vi "Async Data Logger.vi"(8 "error in (no error)":errorcluster, 10 "Log File Ref.":refnum<file>, 11 "User Event In":refnum<user-event>) -> (0 "error out":errorcluster)   [LabVIEW 2024, in "devicePowerSequencerCoreLogic.lvlib"]
doc: "<b> Asynchronous Logger </b> logs the measured data as they are generated. Runs independent of core logic.."
uses:
  devicePowerSequencerCoreLogic.lvlib
  dataLogger/dataLogger.lvlib
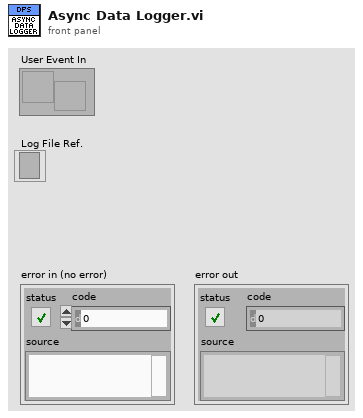
[diagram p1: front panel]
types:
  T1 = cluster{"Measured Data":cluster{"Voltage":dbl[], "Current":dbl[]}[], "Measurment Size":i32[], "Log File Ref.":refnum<file>, "First Call?":bool, "Measure Complete?":bool}
  T2 = enum16{"open", "replace", "create", "open or create", "replace or create", "replace or create with confirmation"}
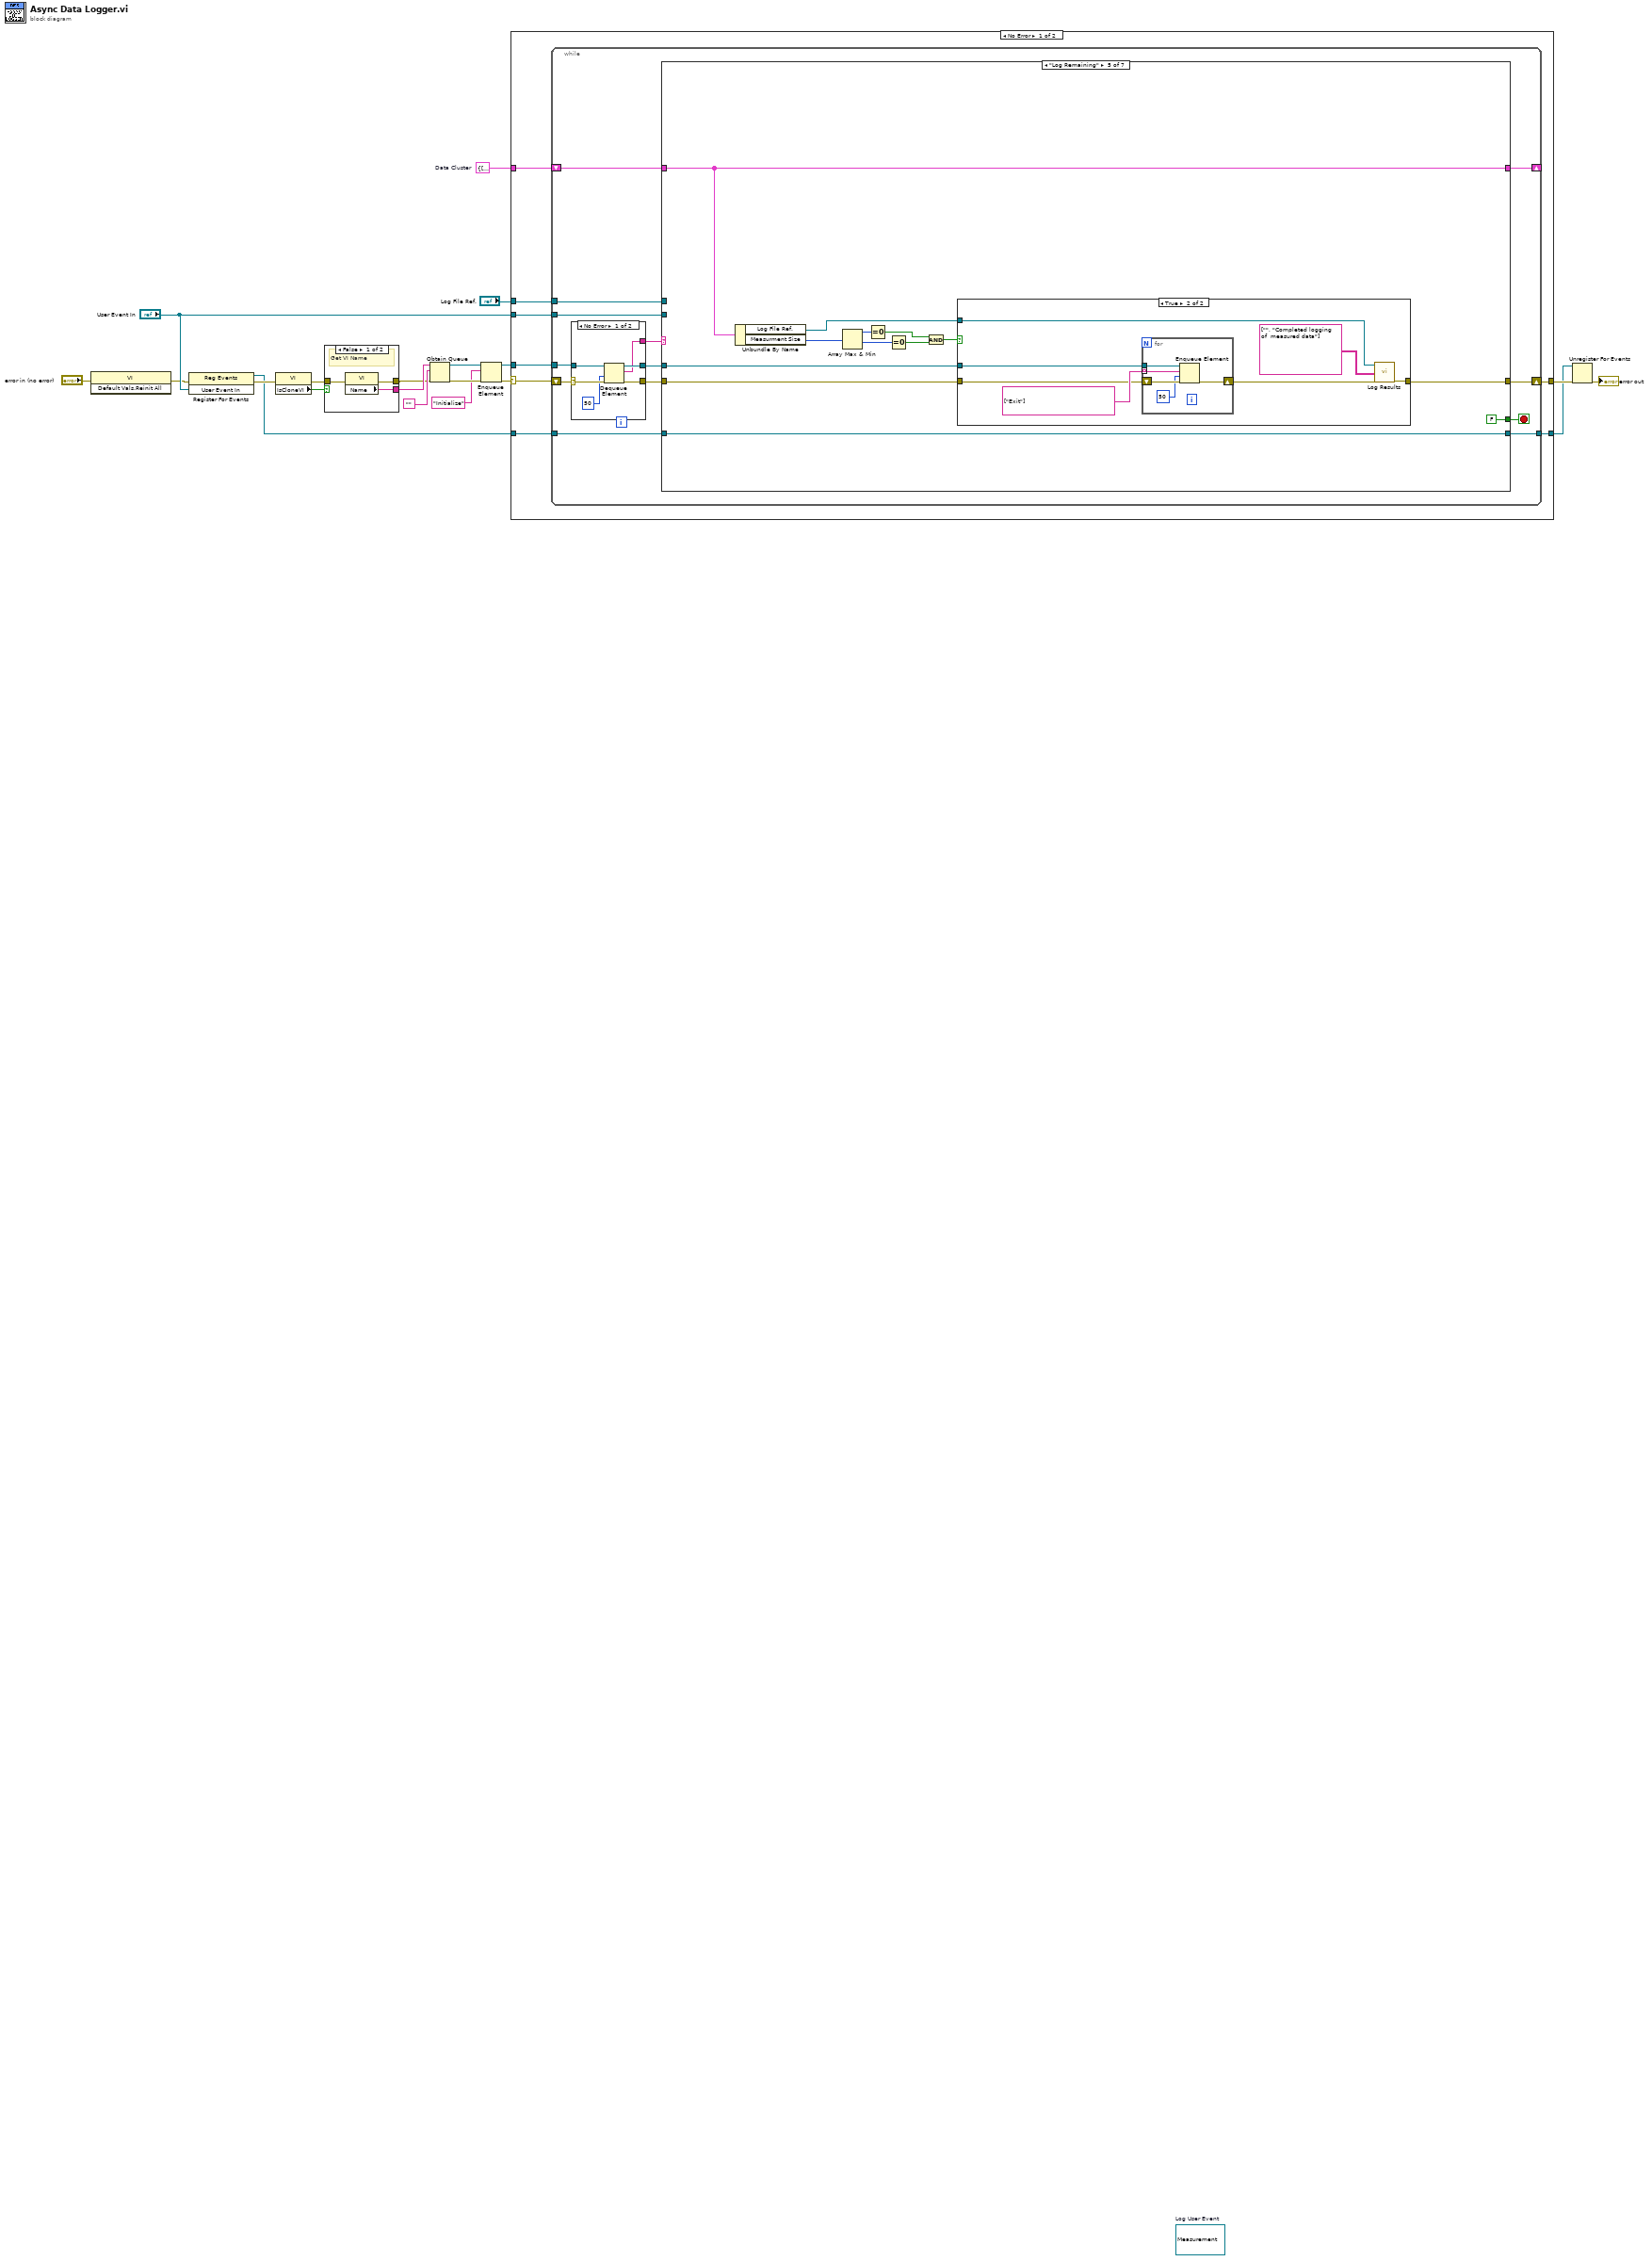
[diagram p0: block diagram]
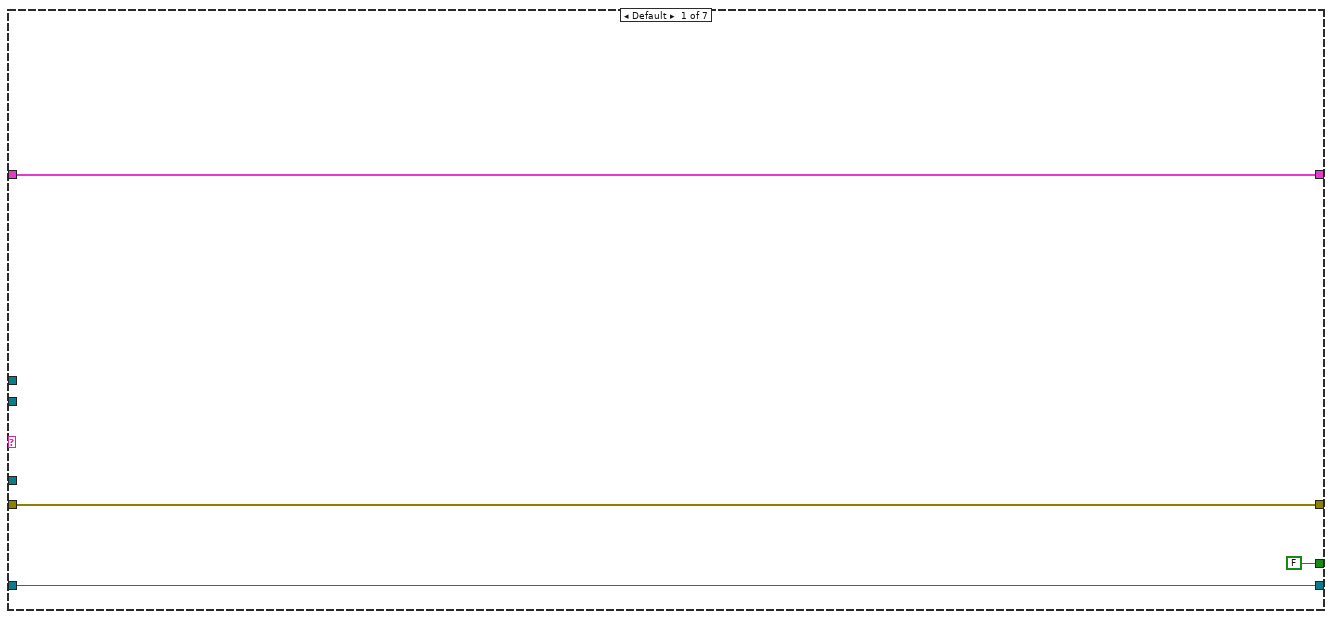
[diagram p2: hidden frame]
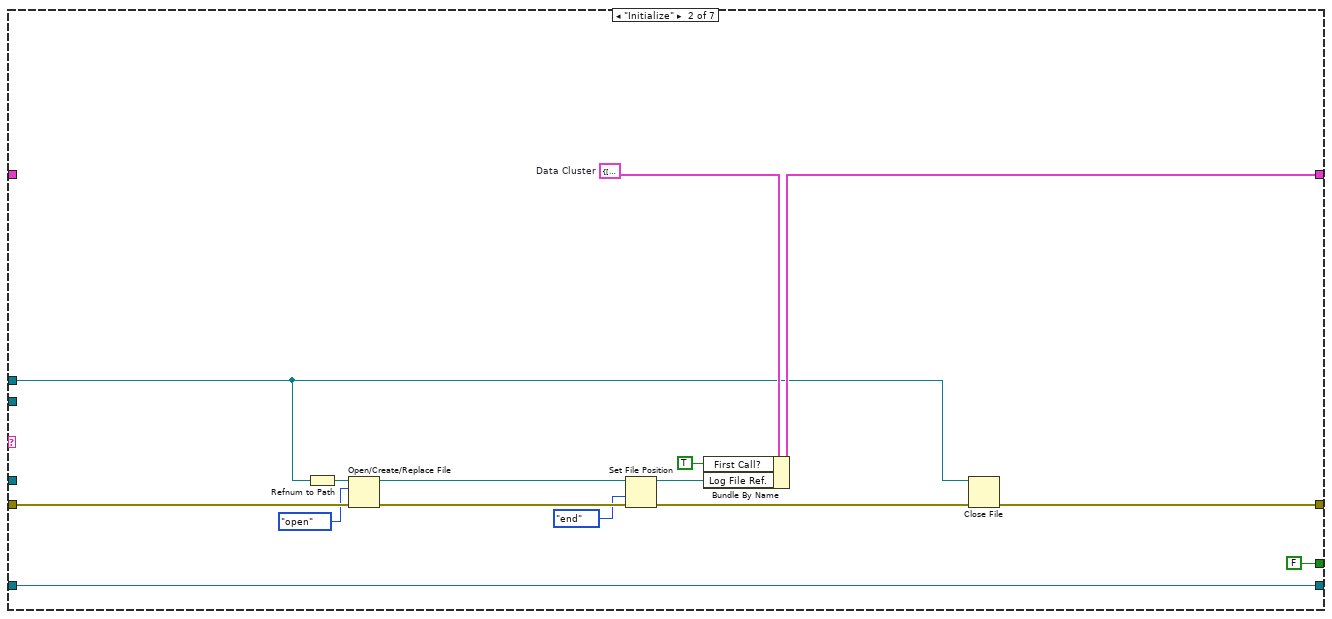
[diagram p3: hidden frame]
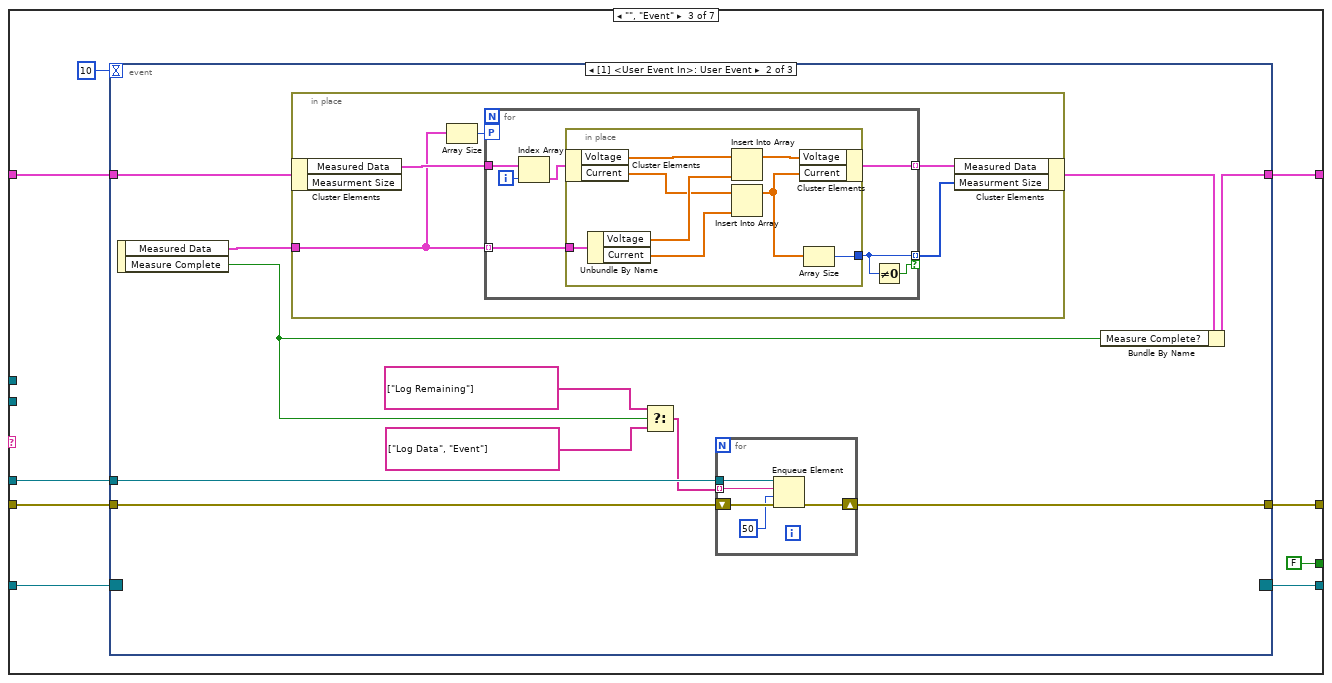
[diagram p4: hidden frame]
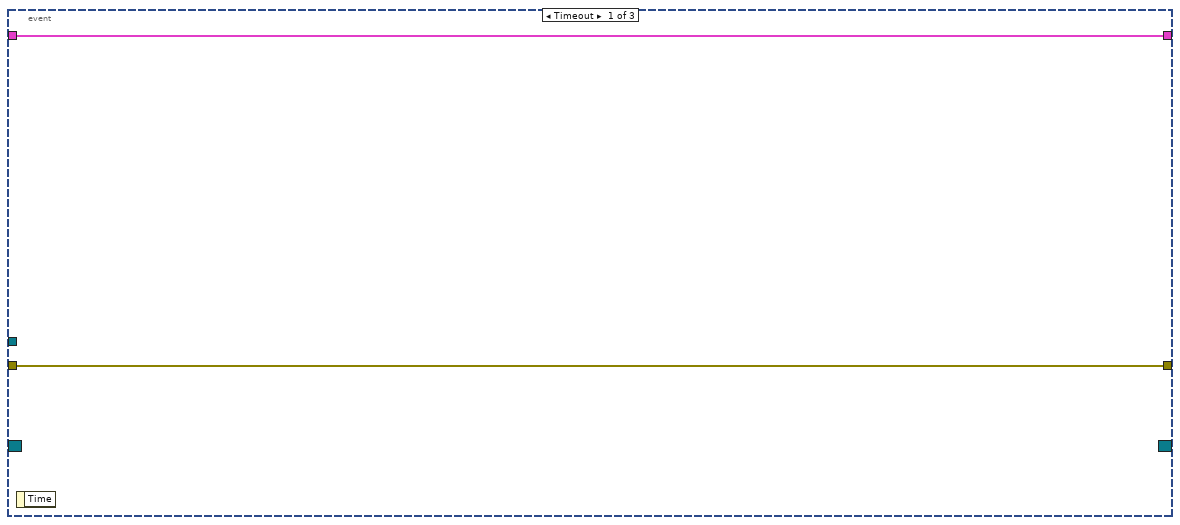
[diagram p5: hidden frame]
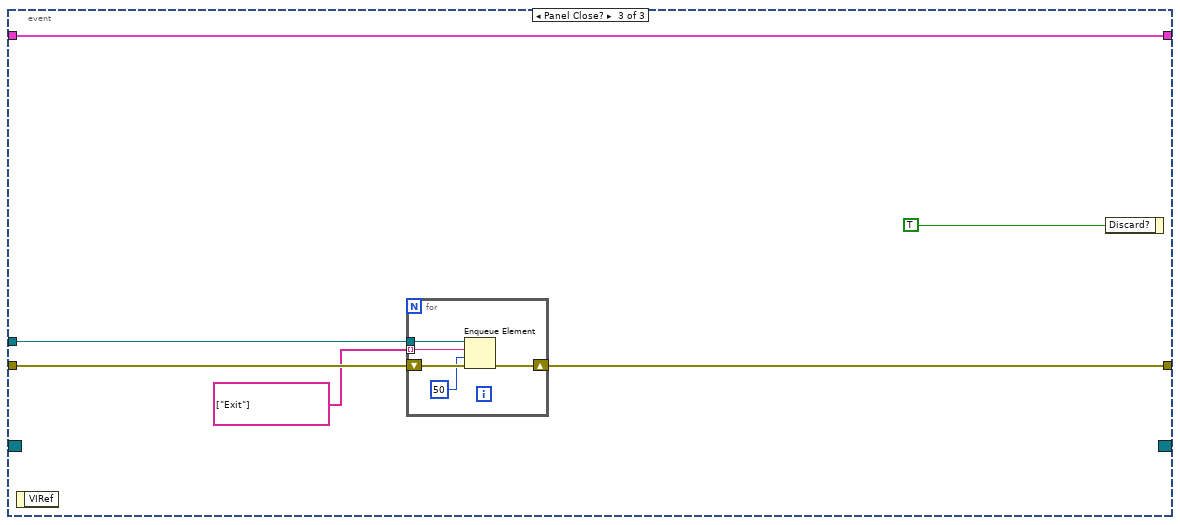
[diagram p6: hidden frame]
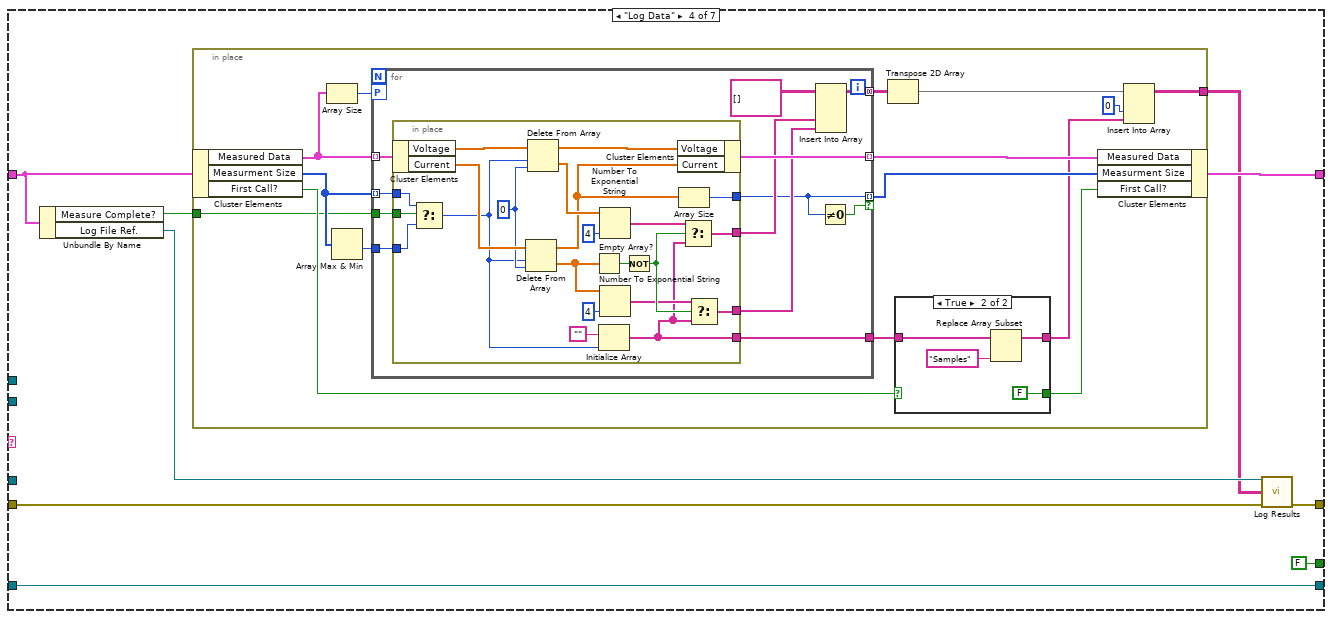
[diagram p7: hidden frame]
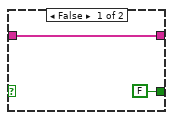
[diagram p8: hidden frame]
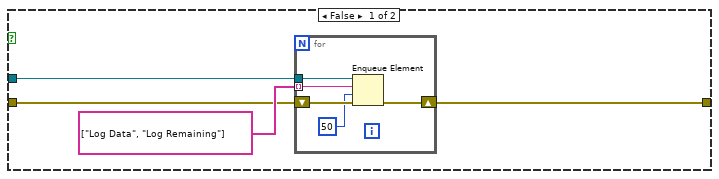
[diagram p9: hidden frame]
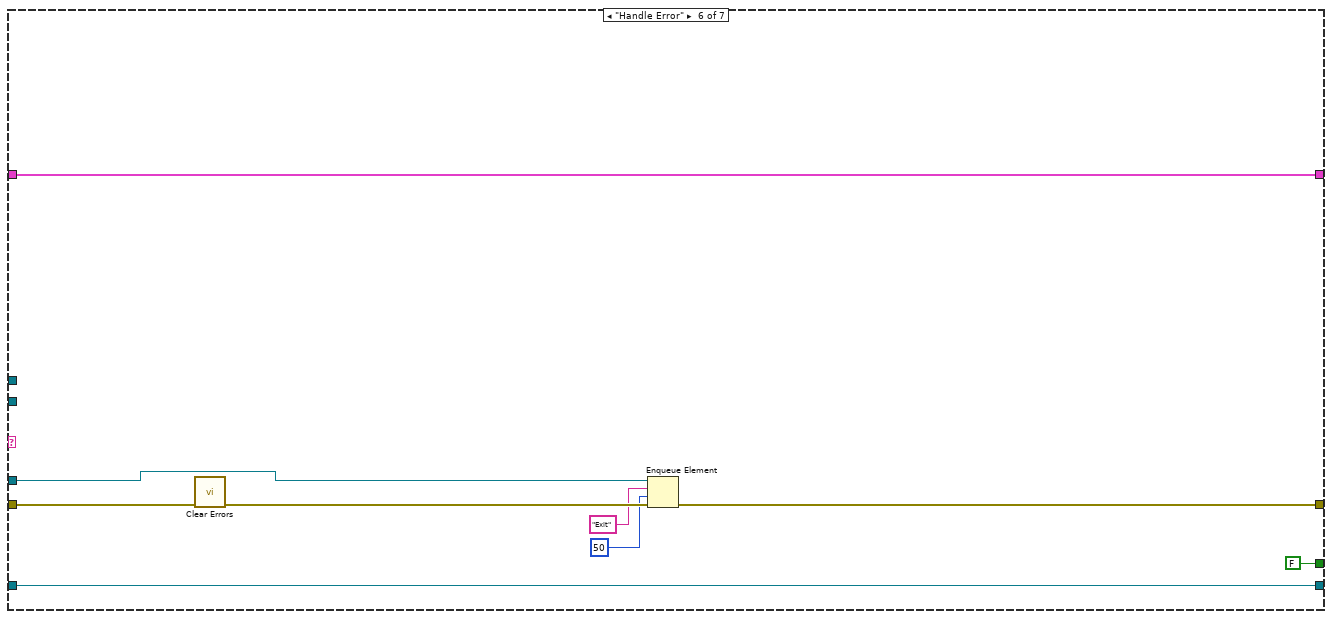
[diagram p10: hidden frame]
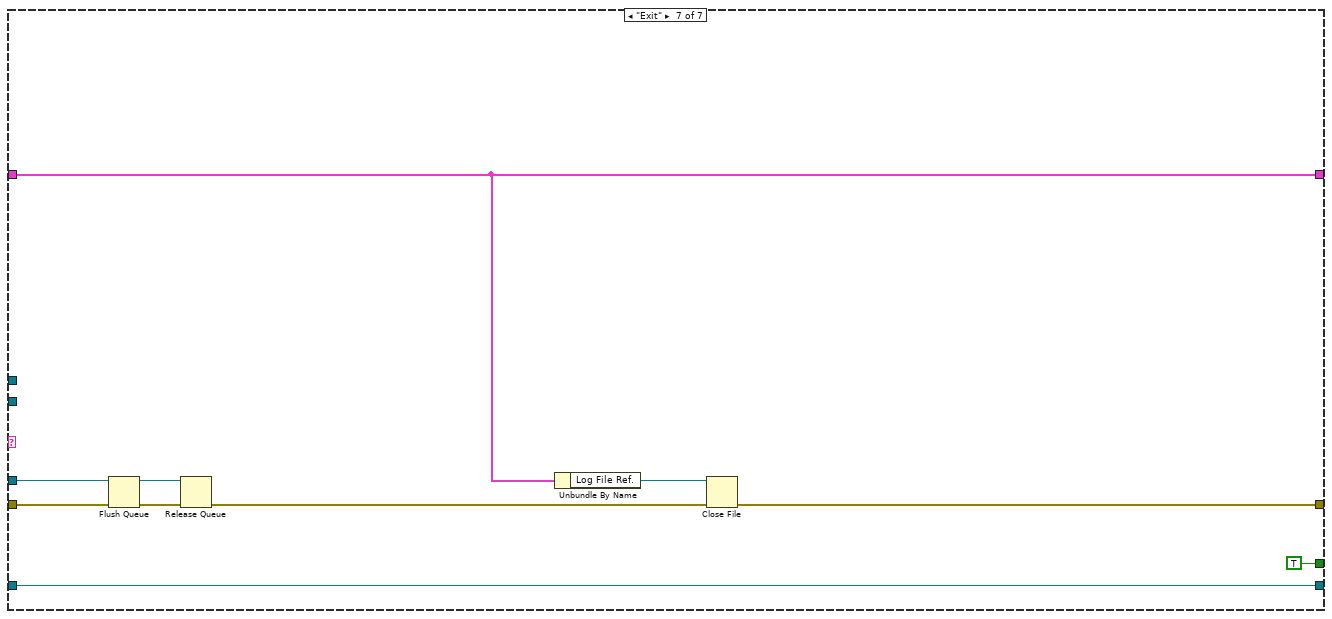
[diagram p11: hidden frame]
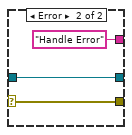
[diagram p12: hidden frame]
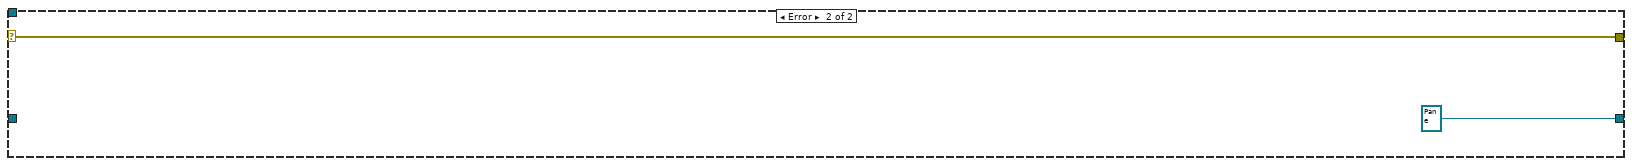
[diagram p13: hidden frame]
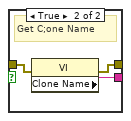
[diagram p14: hidden frame]
diagram:
  (unwired) refnum<user-event> refnum  # Log User Event
  w2 = T1 {"Measured Data"=[], "Measurment Size"=[], "Log File Ref."=refnum, "First Call?"=FALSE, "Measure Complete?"=FALSE}  # Data Cluster
  n1 = invoke class="VI" method="Default Vals.Reinit All"(error in="error in (no error)") -> (error out=w3:errorcluster)  [unwired: 2 in, 2 out]
  n2 = register-events(error in=w3, "User Event In") -> (reference out=w16:refnum<event-registration>, error out=w17:errorcluster)  [unwired: 1 in]
  n3 = property class="VI"(error in=w17) -> (error out=w19:errorcluster, "IsCloneVI"=w5:bool)  [unwired: 1 in, 1 out]
  n4 = case shown="False" w5 {
    tunnel: [w23 w25] -> w10
    tunnel: [w22 w24] -> w11
    tunnel: w19 -> [w21 w26]
    frame False {
      # "Get VI Name"
      n5 = property class="VI"(error in=w21) -> (error out=w23:errorcluster, "Name"=w22:string)  [unwired: 1 in, 1 out]
    }
    frame True {
      # "Get C;one Name"
      n6 = property class="VI"(error in=w26) -> (error out=w25:errorcluster, "Clone Name"=w24:string)  [unwired: 1 in, 1 out]
    }
  }
  n7 = Obtain Queue(name (unnamed)=w11, element data type="" ("Empty String Constant"), error in (no error)=w10) -> (queue out=w14:refnum<queue>, error out=w15:errorcluster)  [unwired: 2 in, 1 out]
  n8 = Enqueue Element(queue=w14, element="Initialize", error in (no error)=w15) -> (queue out=w8:refnum<queue>, error out=w9:errorcluster)  [unwired: 1 in, 1 out]
  n9 = case shown="No Error" w9 {
    selector: w9 -> [w32 w252]
    tunnel: [w34 w252] -> w20
    tunnel: w16 -> [w33 _]
    tunnel: w8 -> [w31 _]
    tunnel: w2 -> [w30 _]
    tunnel: [w29 refnum<event-registration> refnum ("Event Registration Refnum")] -> w6
    tunnel: "User Event In" -> [w28 _]
    tunnel: "Log File Ref." -> [w27 _]
    frame No Error {
      n10 = while {
        shift-right: [w47] -> w34
        shift-left: w32 -> [w44]
        tunnel: w33 -> [w46]
        shift-right: [w40] -> _
        shift-left: w30 -> [w45]
        tunnel: w31 -> [w42]
        tunnel: [w38] -> w29
        tunnel: w28 -> [w36]
        tunnel: w27 -> [w35]
        stop <- w37 stop-if-true
        n11 = case shown="No Error" w44 {
          selector: w44 -> [w247 w250]
          tunnel: [w246 w250] -> w43
          tunnel: w42 -> [w245 w249]
          tunnel: [w244 w249] -> w39
          tunnel: [w243 "Handle Error"] -> w41
          frame No Error {
            n12 = Dequeue Element(queue=w245, timeout in ms (-1)=50, error in (no error)=w247) -> (queue out=w244:refnum<queue>, element=w243:string, error out=w246:errorcluster)  [unwired: 1 out]
          }
          frame Error {
          }
        }
        n13 = case shown="\"Log Remaining\"" w41 {
          tunnel: [w49 w54 w74 w132 w193 w226 w240] -> w47
          tunnel: w43 -> [w49 w65 w73 w131 w194 w228 w236]
          tunnel: w46 -> [w50 w66 w72 w133 w201 w230 w241]
          tunnel: w45 -> [w51 _ w71 w130 w200 w231 w239]
          tunnel: [w51 w64 w70 w129 w200 w231 w239] -> w40
          tunnel: w39 -> [_ _ w69 _ w192 w225 w237]
          tunnel: [w50 w66 w68 w133 w201 w230 w241] -> w38
          tunnel: [FALSE FALSE FALSE FALSE FALSE FALSE TRUE] -> w37
          tunnel: w36 -> [_ _ _ _ _ _ _]
          tunnel: w35 -> [_ w53 _ _ _ _ _]
          frame Default {
          }
          frame "Initialize" {
            w55 = T1 {"Measured Data"=[], "Measurment Size"=[], "Log File Ref."=refnum, "First Call?"=FALSE, "Measure Complete?"=FALSE}  # Data Cluster
            n14 = Refnum to Path(1:w53) -> (0:w63:path)
            n15 = Open/Create/Replace File(file path (use dialog)=w63, error in=w65, operation (0:open)=T2."open") -> (refnum out=w60:refnum<file>, error out=w58:errorcluster)  [unwired: 3 in, 1 out]
            n16 = Set File Position(refnum=w60, from (0:start)=enum16{"start", "end", "current"}."end", error in=w58) -> (refnum out=w59:refnum<file>, error out=w57:errorcluster)  [unwired: 1 in]
            n17 = Bundle By Name(cluster=w55, "First Call?"=TRUE, "Log File Ref."=w59) -> (w64:T1)
            n18 = Close File(refnum=w53, error in=w57) -> (error out=w54:errorcluster)  [unwired: 1 out]
          }
          frame "", "Event" {
            n19 = event shown="[1] <User Event In>: User Event" {
              selector: w72 -> [_ _ _]
              dyn-events: [_ _ _] -> w68
              timeout: 10 -> [_ _ _]
              tunnel: [w77 w84 w114] -> w74
              tunnel: w73 -> [w77 w85 w117]
              tunnel: w71 -> [w76 w87 w119]
              tunnel: [w76 w79 w119] -> w70
              tunnel: w69 -> [_ w86 w116]
              event Timeout {
                n20 = event-data() -> ()  [unwired: 1 in, 1 out]
              }
              event User Event {
                n21 = event-data() -> ("Measured Data"=w88:cluster{"Voltage":dbl[], "Current":dbl[]}[], "Measure Complete"=w78:bool)  [unwired: 1 in]
                n22 = in-place {
                  in-place-border: w88 -> [w89]
                  n23 = in-place-cluster #1(w87) -> ("Measured Data"=w92:cluster{"Voltage":dbl[], "Current":dbl[]}[])  [unwired: 1 out]
                  n24 = Array Size(array=w89) -> (size(s)=w93:i32)
                  n25 = for {
                    tunnel: w92 -> [w98]
                    workers-P: w93 -> [_]
                    tunnel: w89 -> [w100] mode=indexing
                    tunnel: [w99] -> w91 mode=indexing
                    tunnel: [w95] -> w90 mode=indexing if=w94
                    i -> [w97]
                    n26 = Index Array(array=w98, index=w97) -> (element=w96:cluster{"Voltage":dbl[], "Current":dbl[]})
                    n27 = in-place {
                      in-place-border: w100 -> [w107]
                      in-place-border: [w102] -> w95
                      n28 = in-place-cluster #2(w96) -> ("Voltage"=w108:dbl[], "Current"=w105:dbl[])
                      n29 = Unbundle By Name(w107) -> ("Voltage"=w106:dbl[], "Current"=w103:dbl[])
                      n30 = Insert Into Array(array=w108, new element=w106) -> (w104:dbl[])  [unwired: 1 in]
                      n31 = Insert Into Array(array=w105, new element=w103) -> (w101:dbl[])  [unwired: 1 in]
                      n32 = in-place-cluster #2("Voltage"=w104, "Current"=w101) -> (w99:cluster{"Voltage":dbl[], "Current":dbl[]})
                      n33 = Array Size(array=w101) -> (size(s)=w102:i32)
                    }
                    n34 = Not Equal To 0?(x=w95) -> (x != 0?=w94:bool)
                  }
                  n35 = in-place-cluster #1("Measured Data"=w91, "Measurment Size"=w90) -> (w83:T1)
                }
                n36 = Select(t=string[] ["Log Remaining"], s=w78, f=string[] ["Log Data", "Event"]) -> (s? t:f=w82:string[])
                n37 = for {
                  shift-right: [w112] -> w84
                  shift-left: w85 -> [w113]
                  tunnel: w86 -> [w111]
                  tunnel: w82 -> [w110] mode=indexing
                  n38 = Enqueue Element(queue=w111, element=w110, timeout in ms (-1)=50, error in (no error)=w113) -> (error out=w112:errorcluster)  [unwired: 2 out]
                }
                n39 = Bundle By Name(cluster=w83, "Measure Complete?"=w78) -> (w79:T1)
              }
              event Panel Close? {
                n40 = event-data() -> ()  [unwired: 1 in, 1 out]
                n41 = for {
                  shift-right: [w123] -> w114
                  shift-left: w117 -> [w124]
                  tunnel: w116 -> [w122]
                  tunnel: string[] ["Exit"] -> [w121] mode=indexing
                  n42 = Enqueue Element(queue=w122, element=w121, timeout in ms (-1)=50, error in (no error)=w124) -> (error out=w123:errorcluster)  [unwired: 2 out]
                }
                n43 = event-data("Discard?"=TRUE) -> ()  [unwired: 1 in, 1 out]
              }
            }
          }
          frame "Log Data" {
            n44 = Unbundle By Name(w130) -> ("Measure Complete?"=w125:bool, "Log File Ref."=w128:refnum<file>)
            n45 = in-place {
              in-place-border: [w144] -> w127
              in-place-border: w125 -> [w134]
              n46 = in-place-cluster #3(w130) -> ("Measured Data"=w141:cluster{"Voltage":dbl[], "Current":dbl[]}[], "Measurment Size"=w135:i32[], "First Call?"=w138:bool)
              n47 = Array Size(array=w141) -> (size(s)=w140:i32)
              n48 = Array Max & Min(array=w135) -> (min value=w142:i32)  [unwired: 3 out]
              n49 = for {
                tunnel: w142 -> [w166]
                tunnel: w141 -> [w165] mode=indexing
                tunnel: [w164] -> w148 mode=indexing
                tunnel: [w160] -> w145 mode=indexing if=w159
                tunnel: [w158] -> w139
                tunnel: [w163] -> w147 mode=concatenating
                workers-P: w140 -> [_]
                tunnel: w135 -> [w156] mode=indexing
                tunnel: w134 -> [w155]
                n50 = in-place {
                  in-place-border: w166 -> [w170]
                  in-place-border: [w178] -> w162
                  in-place-border: [w177] -> w161
                  in-place-border: [w175] -> w160
                  in-place-border: [w171] -> w158
                  in-place-border: w156 -> [w169]
                  in-place-border: w155 -> [w168]
                  w174 = 0 ("index")
                  n51 = in-place-cluster #4(w165) -> ("Voltage"=w188:dbl[], "Current"=w187:dbl[])
                  n52 = Select(t=w169, s=w168, f=w170) -> (s? t:f=w167:i32)
                  n53 = Delete From Array(array=w187, length=w167, index=w174) -> (deleted portion=w179:dbl[], array with subset deleted=w176:dbl[])
                  n54 = Delete From Array(array=w188, length=w167, index=w174) -> (deleted portion=w181:dbl[], array with subset deleted=w186:dbl[])
                  n55 = Empty Array?(array=w179) -> (empty?=w185:bool)
                  n56 = Initialize Array("", w167) -> (w171:string[])
                  n57 = Number To Exponential String(number=w181, precision (6)=i16 4) -> (E-format string=w180:string[])  [unwired: 2 in]
                  n58 = Number To Exponential String(number=w179, precision (6)=i16 4) -> (E-format string=w182:string[])  [unwired: 2 in]
                  n59 = Not(x=w185) -> (.not. x?=w184:bool)
                  n60 = in-place-cluster #4("Voltage"=w186, "Current"=w176) -> (w164:cluster{"Voltage":dbl[], "Current":dbl[]})
                  n61 = Array Size(array=w176) -> (size(s)=w175:i32)
                  n62 = Select(t=w180, s=w184, f=w171) -> (s? t:f=w178:string[])
                  n63 = Select(t=w182, s=w184, f=w171) -> (s? t:f=w177:string[])
                }
                n64 = Insert Into Array(array=string[][] [], new element #1=w162, new element #2=w161) -> (w163:string[][])  [unwired: 2 in]
                n65 = Not Equal To 0?(x=w160) -> (x != 0?=w159:bool)
              }
              n66 = Transpose 2D Array(2D array=w147) -> (transposed array=w146:string[][])
              n67 = case shown="True" w138 {
                tunnel: w139 -> [w150 w154]
                tunnel: [FALSE FALSE] -> w137
                tunnel: [w150 w151] -> w136
                frame False {
                }
                frame True {
                  n68 = Replace Array Subset(array=w154, new element="Samples" ("new element/subarray")) -> (w151:string[])  [unwired: 1 in]
                }
              }
              n69 = in-place-cluster #3("Measured Data"=w148, "Measurment Size"=w145, "First Call?"=w137) -> (w129:T1)
              n70 = Insert Into Array(array=w146, index (col)=0 ("disabled index (col)"), new element=w136) -> (w144:string[][])  [unwired: 1 in]
            }
            n71 = call "Log Results.vi"("Log File Ref. In"=w128, "Data Input"=w127, "error in"=w131) -> ("error out"=w132:errorcluster)  [unwired: 10 in, 2 out]
          }
          frame "Log Remaining" {
            n72 = Unbundle By Name(w200) -> ("Log File Ref."=w189:refnum<file>, "Measurment Size"=w199:i32[])
            n73 = Array Max & Min(array=w199) -> (max value=w197:i32, min value=w198:i32)  [unwired: 2 out]
            n74 = Equal To 0?(x=w197) -> (x = 0?=w195:bool)
            n75 = Equal To 0?(x=w198) -> (x = 0?=w196:bool)
            n76 = And(x=w195, y=w196) -> (x .and. y?=w191:bool)
            n77 = case shown="True" w191 {
              tunnel: w194 -> [w204 w216]
              tunnel: [w203 w213] -> w193
              tunnel: w192 -> [w202 w215]
              tunnel: w189 -> [_ w212]
              frame False {
                n78 = for {
                  shift-right: [w209] -> w203
                  shift-left: w204 -> [w210]
                  tunnel: w202 -> [w208]
                  tunnel: string[] ["Log Data", "Log Remaining"] -> [w207] mode=indexing
                  n79 = Enqueue Element(queue=w208, element=w207, timeout in ms (-1)=50, error in (no error)=w210) -> (error out=w209:errorcluster)  [unwired: 2 out]
                }
              }
              frame True {
                n80 = for {
                  shift-right: [w221] -> w214
                  shift-left: w216 -> [w222]
                  tunnel: w215 -> [w220]
                  tunnel: string[] ["Exit"] -> [w219] mode=indexing
                  n81 = Enqueue Element(queue=w220, element=w219, timeout in ms (-1)=50, error in (no error)=w222) -> (error out=w221:errorcluster)  [unwired: 2 out]
                }
                n82 = call "Log Results.vi"("Log File Ref. In"=w212, "Data Input"=string[][] [[""], ["Completed logging of  measured data"]], "error in"=w214) -> ("error out"=w213:errorcluster)  [unwired: 10 in, 2 out]
              }
            }
          }
          frame "Handle Error" {
            n83 = call <vilib>:"Clear Errors.vi"("error in (no error)"=w228) -> ("error out"=w227:errorcluster)  [unwired: 5 in, 1 out]
            n84 = Enqueue Element(queue=w225, element="Exit", timeout in ms (-1)=50, error in (no error)=w227) -> (error out=w226:errorcluster)  [unwired: 2 out]
          }
          frame "Exit" {
            n85 = Flush Queue(queue=w237, error in (no error)=w236) -> (queue out=w234:refnum<queue>, error out=w235:errorcluster)  [unwired: 1 out]
            n86 = Release Queue(queue=w234, error in (no error)=w235) -> (error out=w233:errorcluster)  [unwired: 1 in, 2 out]
            n87 = Unbundle By Name(w239) -> ("Log File Ref."=w232:refnum<file>)
            n88 = Close File(refnum=w232, error in=w233) -> (error out=w240:errorcluster)  [unwired: 1 out]
          }
        }
      }
    }
    frame Error {
    }
  }
  n89 = Unregister For Events(event registration refnum=w6, error in=w20) -> (error out=→"error out":errorcluster)
